vi "FX07.vi"(11 "Variables and Memory in":T1 {"GFX" format="%02x"}) -> (3 "Variables and Memory out":T1 {"GFX" format="%02x"})   [LabVIEW 2021]
uses:
  Controls/ClusterF.ctl
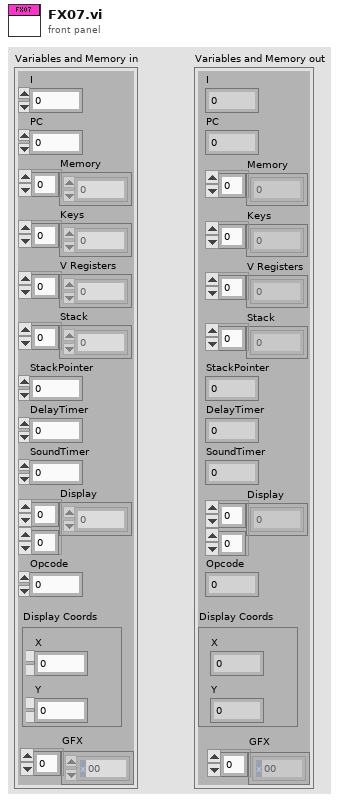
[diagram p1: front panel]
types:
  T1 = typedef "ClusterF.ctl" = cluster{"I":u16, "PC":u16, "Memory":u8[], "Keys":u8[], "V Registers":u8[], "Stack":u16[], "StackPointer":u16, "DelayTimer":u8, "SoundTimer":u8, "Display":u8[][], "Opcode":u16, "Display Coords":cluster{"X":u8, "Y":u8}, "GFX":u8[]}
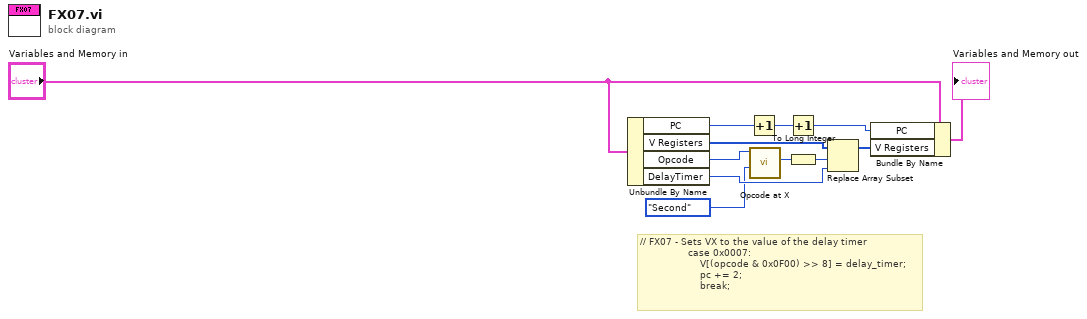
[diagram p0: block diagram]
diagram:
  # "// FX07 - Sets VX to the value of the delay timer\n                case 0x0007:\n                    V[(opcode & 0x0F00) >> 8] = delay_timer;\n                    pc += 2;\n                    break;"
  n1 = Unbundle By Name("Variables and Memory in") -> ("PC"=w3:u16, "V Registers"=w6:u8[], "Opcode"=w7:u16, "DelayTimer"=w10:u8)
  n2 = Increment(x=w3) -> (x+1=w4:u16)
  n3 = call "Opcode at X.vi"("X Position"=enum16{"First", "Second", "Third", "Fourth"}."Second", "Opcode"=w7) -> ("Opcode at X Position (U8)"=w8:u8)  [unwired: 9 in]
  n4 = Increment(x=w4) -> (x+1=w5:u16)
  n5 = To Long Integer(number=w8) -> (32bit integer=w11:i32)
  n6 = Replace Array Subset(array=w6, new element=w10, index=w11) -> (w12:u8[])
  n7 = Bundle By Name(cluster="Variables and Memory in", "PC"=w5, "V Registers"=w12) -> (→"Variables and Memory out":T1)
